vi "Sample Transfer Close All Containers.vi"(8 "error in (no error)":errorcluster, 11 "cRIO-CO2 in":refnum<class "cRIO-CO2.lvclass">) -> (0 "error out":errorcluster, 3 "cRIO-CO2 out":refnum<class "cRIO-CO2.lvclass">)   [LabVIEW 2015, in "cRIO-Carbondioxide.lvlib" / "cRIO-CO2.lvlib" / "cRIO-CO2.lvclass"]
uses:
  cRIO-CO2.lvclass
  Controls/Sample Line State Enumerator.ctl
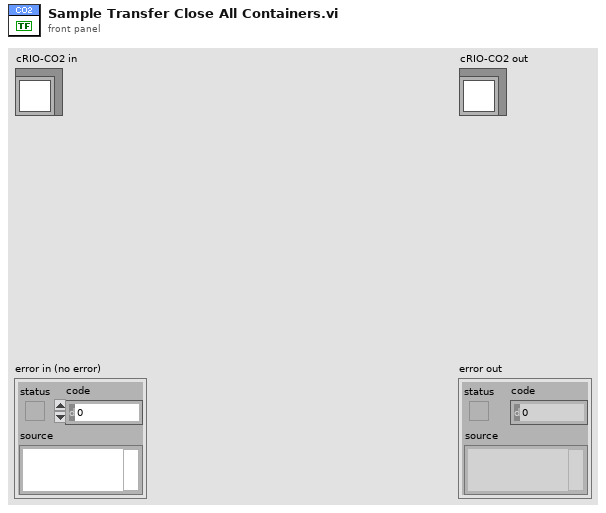
[diagram p1: front panel]
types:
  T1 = typedef "Sample Line State Enumerator.ctl" = enum16{"All lines closed", "Sample line 1.", "Sample line 2.", "Sample line 3.", "Sample line 4.", "Sample line 5.", "Out of range"}
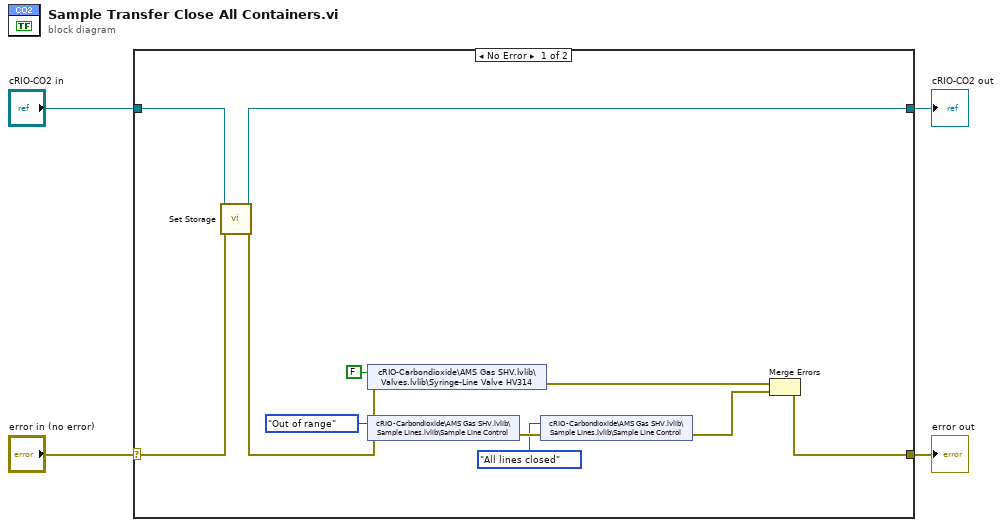
[diagram p0: block diagram]
diagram:
  n1 = case shown="No Error" "error in (no error)" {
    selector: "error in (no error)" -> [w7 w17]
    tunnel: [w13 w17] -> w3
    tunnel: [w8 w16] -> w1
    tunnel: "cRIO-CO2 in" -> [w9 w16]
    frame No Error {
      n2 = call "Set Storage.vi"("error in (no error)"=w7, "cRIO-CO2 in"=w9) -> ("error out"=w6:errorcluster, "cRIO-CO2 out"=w8:refnum<class "cRIO-CO2.lvclass">)  [unwired: 8 in]
      n3 = shared-variable "cRIO-Carbondioxide\\AMS Gas SHV.lvlib\\Valves.lvlib\\Syringe-Line Valve HV314"(FALSE ("Syringe-Line Valve HV314"), error in=w6) -> (error out=w14:errorcluster)
      n4 = shared-variable "cRIO-Carbondioxide\\AMS Gas SHV.lvlib\\Sample Lines.lvlib\\Sample Line Control"(Sample_Line_State_Enumerator."Out of range" ("Sample Line Control"), error in=w6) -> (error out=w12:errorcluster)
      n5 = shared-variable "cRIO-Carbondioxide\\AMS Gas SHV.lvlib\\Sample Lines.lvlib\\Sample Line Control"(Sample_Line_State_Enumerator."All lines closed" ("Sample Line Control"), error in=w12) -> (error out=w5:errorcluster)
      n6 = Merge Errors(w14, w5) -> (w13:errorcluster)
    }
    frame Error {
    }
  }
  "error out" <- w3
  "cRIO-CO2 out" <- w1
